vi "Get Menu Commands.vi"(8 "error in (no error)":errorcluster, 9 "Active Build Configuration":string, 10 "Selected Items":string[][](array[string]), 11 "Build Package Item in":refnum<class "Build Package Item.lvclass">) -> (0 "error out":errorcluster, 2 "Menu":string[](array[string]))   [LabVIEW 2019, in "VIPM.lvlib" / "Build Package Item.lvclass"]
uses:
  Build Package Item.lvclass
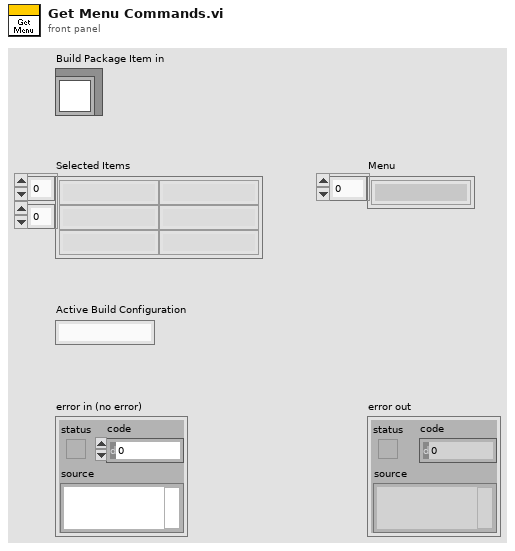
[diagram p1: front panel]
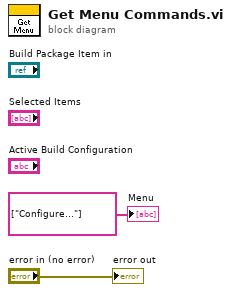
[diagram p0: block diagram]
diagram:
  "error out" <- "error in (no error)"
  "Menu" <- string[] ["Configure..."] ("Menu")
